vi "Main_PXI_v1.0.vi"() -> ()   [LabVIEW 2018]
doc: "Main VI for the controls"
uses:
  components/pmcl dynamic signal analyzer/Controls/DSA excitation specs.ctl
  components/pmcl dynamic signal analyzer/Controls/DSA cycle specs.ctl
  Typedefs/StateDef_Enum.ctl
  <vilib>/Simulation/Scripting/Companion Diagram/SimConfigNode/SimParams.ctl
  <vilib>/Simulation/Scripting/Companion Diagram/SimConfigNode/_simSolvers.ctl
  <vilib>/Simulation/Implementation/Shared/SIMSCR Execution Mode.ctl
  <vilib>/Platform/TimedLoop/XDataNode/timing_clust.ctl
  <vilib>/Platform/TimedLoop/XDataNode/nitl_modes.ctl
  <vilib>/Platform/TimedLoop/XDataNode/wakeup.ctl
  <vilib>/Simulation/Param Hierarchy/Typedefs/SIMPH Param Control Actions.ctl
  <vilib>/Simulation/Implementation/Shared/SIM limit type.ctl
  <vilib>/Simulation/Scripting/Editor Utilities/SIM subVI tag data.ctl
  <vilib>/Simulation/Scripting/Editor Utilities/SIM subVI execution type.ctl
  <vilib>/Simulation/Implementation/Shared/NILVSim_ParamChanged.vi
  <vilib>/Simulation/Implementation/Shared/NILVSim_FinishedLate.vi
  <vilib>/Simulation/Implementation/Shared/NILVSIM_BeginStep.vi
  <vilib>/DAQmx/read.llb/DAQmx Read.vi
  <vilib>/DAQmx/read.llb/DAQmx Read (Analog 1D DBL NChan 1Samp).vi
  <vilib>/Simulation/Utility/Implementation/SIM SimulationParams.vi
  <vilib>/Simulation/ContinuousLinear/Implementation/NILVSim Integrator new.llb/SIM Integrator distributor (scalar).vi
  <vilib>/Simulation/Implementation/Shared/SIM Fire Discrete SubVI.vi
  <vilib>/Simulation/ContinuousLinear/Implementation/NILVSim Transfer Function Direct.llb/SIM Transfer Function Direct (SISO).vi
  <vilib>/DAQmx/write.llb/DAQmx Write (Analog DBL 1Chan 1Samp).vi
  <vilib>/Simulation/Utility/Implementation/SIM Halt.vi
  <vilib>/Simulation/SignalArithmetic/Implementation/NILVSim Gain.llb/SIM Gain (scalar).vi
  <vilib>/Simulation/ContinuousLinear/Implementation/NILVSim Integrator new.llb/SIM Integrator collector (scalar).vi
  <vilib>/Simulation/Implementation/Shared/NILVSim_Manager.vi
  <vilib>/Utility/error.llb/Clear Errors.vi
  <vilib>/Simulation/Implementation/Shared/NILVSim_FinalizeModel.vi
  <vilib>/Simulation/Utility/Implementation/NILVSim SimulationParams (core).vi
  <vilib>/Simulation/Implementation/Shared/SIM Fire Discrete SubVI (Core).vi
  <vilib>/DAQmx/create/channels.llb/DAQmx Create Channel (AO-Voltage-Basic).vi
  <vilib>/DAQmx/create/channels.llb/DAQmx Create Channel (AI-Voltage-Basic).vi
  <vilib>/Simulation/Implementation/Shared/SIM Unbundle Sim Info.vi
  <vilib>/Simulation/Implementation/Shared/SIMSH Read Queue.vi
  <vilib>/Simulation/Implementation/Shared/NILVSim_Initialize.vi
  <vilib>/DAQmx/miscellaneous.llb/DAQmx Fill In Error Info.vi
  <vilib>/Simulation/Utility/Implementation/NILVSim Get Time and IsAcceptedStep.vi
  <vilib>/Simulation/Implementation/Shared/NILVSim_GetModelError.vi
  <vilib>/Simulation/Implementation/Shared/SIM Bundle Sim Info.vi
  <vilib>/Simulation/Scripting/Companion Diagram/SimConfigNode/SimDog.xnode
  <vilib>/Platform/TimedLoop/XDataNode/XDataNode.xnode
  <vilib>/Simulation/Implementation/XNodeFramework/SimXNode/SimX.xnode
  Components/Timing/Timing.lvlib
  <vilib>/Platform/TimedLoop/XDataNode/XDNodeRunTimeDep.lvlib
  <vilib>/Analysis/NI_AALPro.lvlib
  <vilib>/ptbypt/NI_PtbyPt.lvlib
  <vilib>/Simulation/ContinuousLinear/Implementation/NILVSim Integrator new.llb/SIM Integrator (scalar).vi
  <vilib>/Simulation/Implementation/Shared/NI_SIM_Implementation.lvlib
panel:
  in  "System Stop Button":bool
  in  "Pause chart?":bool
  in  "Controller Params":enum32{"Page 1"}(tab)
  in  "Kp":dbl=1.0 min=0.0
  in  "Controller On?":bool
  out "Status":string
  in  "Ref. Gen.":enum32{"Analog In", "Manual", "Wave Gen", "DSA"}(tab)=enum."Wave Gen"
  in  "Ref. cmd.":dbl(slide) step=1.0 scale=-10.0..10.0 scale format="%#.1f"
  in  "Signal Cluster":T1={"phase"=0.0, "amplitude"=1.0, "frequency"=1.0, "offset"=1.0, "Signal"=enum."Square"} {"offset" format="%0.2f"; "frequency" format="%0.2f"; "amplitude" format="%0.2f"; "phase" format="%0.2f"}
  in  "Frequency\nResponse":enum16{"Plant", "RR", "CL"}(ring)
  out "DSA \nRunning?":bool
  in  "Stop \nDSA":bool
  in  "Start \nDSA":bool
  in  "DSA excitation specs":T2={"Initial Freq. [Hz]"=10.0, "Final Freq. [Hz]"=999.0, "# pts. in interval"=50, "Samping Time [s]"=0.001, "Amplitude [V]"=1.0, "Offset [V]"=0.0, "Freq Units (F: rad/s, T: Hz)"=TRUE}
  in  "Cycle Specs":T3={"Cycles To \nSettle (M)"=5, "Cycles To \nCalculate (N)"=10}
  in  "Loop Timing":enum32{"CD&Sim", "Ref. gen", "UI"}(tab)
  out "# Finished\nLate counter":dbl
  in  "CD&Sim\nLoop Rate (Hz)":dbl=10000.0 format="%#_4p"
  out "# Finished\nLate counter":dbl
  in  "Ref. Gen.\nLoop Rate (Hz)":dbl=10000.0 format="%#_4p"
  in  "UI Loop rate (Hz)":dbl=1000.0 format="%#_6p"
  in  "Display Waveforms":enum32{"Controller Signals", "DSA "}(tab)
  out "Control Effort":dbl(graph)
  out "Waveform Chart":cluster{"Double":dbl, "Numeric":dbl}(graph)
  out "Phase Bode Plot":cluster{dbl[], dbl[]}(graph)
  out "Magnitude Bode Plot":cluster{dbl[], dbl[]}(graph)
  out "DSA Signals":cluster{"Double":dbl, "Double":dbl}(graph)
  # "Connect the Reference Signal \nto C/AI 1 of the myRIO."
  # "Pinout Config.:\nPort C/AI0 : Plant output being read           by the myRIO.\nPort C/AI1 : Reference signal for the control loop.\nPort C/AO0 : Control effort signal to the plant."
  # "Control Loop Timing"
  # "Ref.  Gen. Loop Timing"
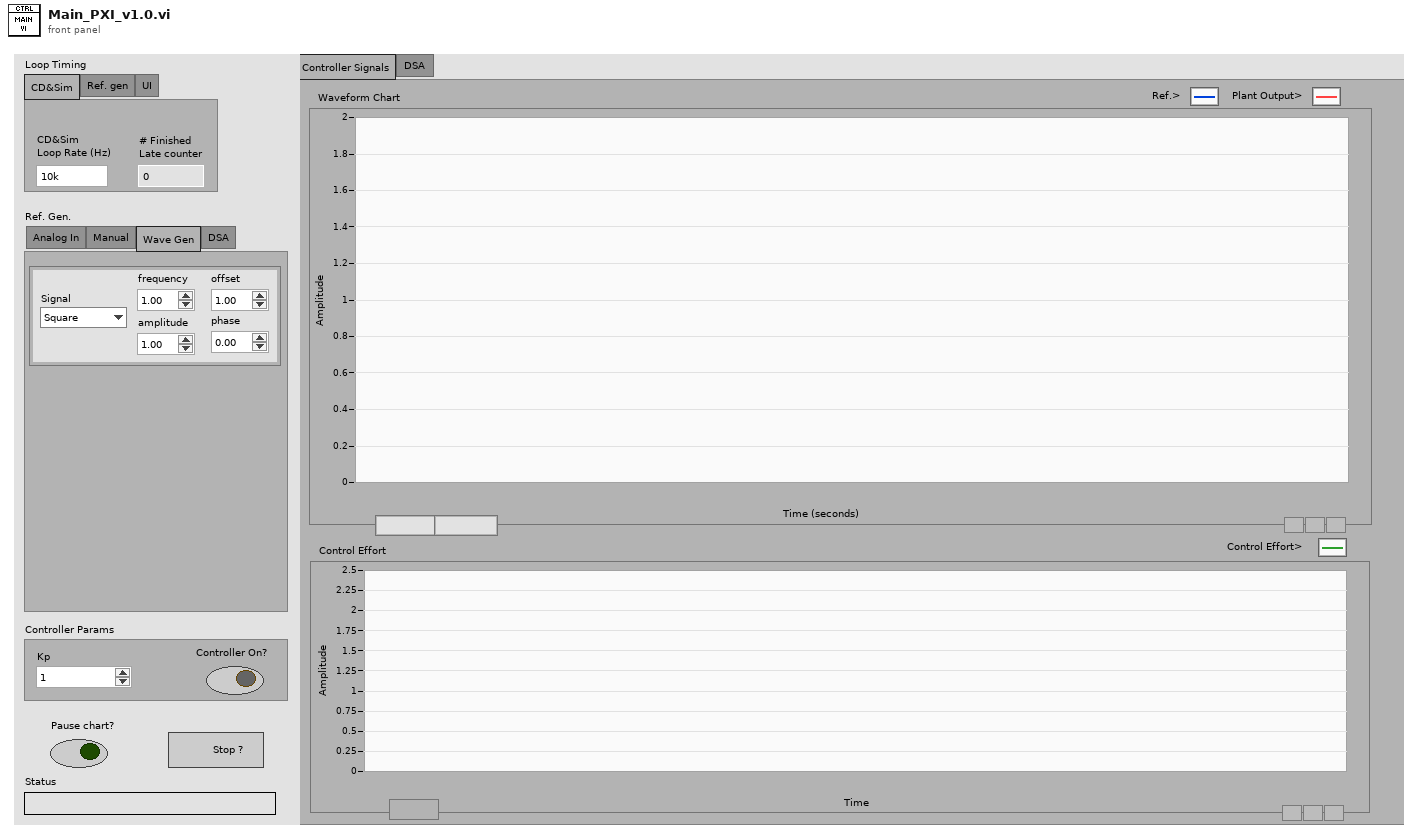
[diagram p1: front panel]
types:
  T1 = cluster{"phase":dbl, "amplitude":dbl, "frequency":dbl, "offset":dbl, "Signal":enum16{"Sine", "Square", "Sawtooth"}}
  T2 = typedef "DSA excitation specs.ctl" = cluster{"Initial Freq. [Hz]":dbl, "Final Freq. [Hz]":dbl, "# pts. in interval":i16, "Samping Time [s]":dbl, "Amplitude [V]":dbl, "Offset [V]":dbl, "Freq Units (F: rad/s, T: Hz)":bool}
  T3 = typedef "DSA cycle specs.ctl" = cluster{"Cycles To \nSettle (M)":i16, "Cycles To \nCalculate (N)":i16}
  T4 = typedef "StateDef_Enum.ctl" = enum16{"Initialize", "Wait", "Shutdown"}
  T5 = typedef "XDNodeRunTimeDep.lvlib/timing_clust.ctl" = cluster{"Expected End [f-1]":u64, "Actual End [f-1]":u64, "Finished Late? [f-1]":bool, "Expected End [i-1]":u64, "Actual End [i-1]":u64, "Finished Late? [i-1]":bool, "Expected Start [i]":u64, "Actual Start [i]":u64, "Expected Start [f]":u64, "Actual Start [f]":u64, "Source Name":string, "Structure Name":string, "Period":i64, "Deadline":i64, "Offset":i64, "Start":i64, "Priority":i32, "Timeout":i32, "Mode":T6, "Wakeup Reason":T7, "Error":errorcluster, "Source Type":string, "Secondary Source Type":string, "Global End Time":u64, "Global Start Time":u64, "Frame Duration":u64, "Iteration Duration":u64, "Assigned CPU":i32, "I/O Scan Engine Mode":u32}
  T6 = typedef "XDNodeRunTimeDep.lvlib/nitl_modes.ctl" = enum32{"No Change", "Process missed periods, maintain original phase", "Discard missed periods, maintain original phase", "Process missed periods, ignore original phase", "Discard missed periods, ignore original phase"}
  T7 = typedef "XDNodeRunTimeDep.lvlib/wakeup.ctl" = enum32{"Normal", "Aborted", "Asynchronous wakeup", "Timing source error", "Timed loop error", "Timeout"}
  T8 = cluster{"Analog In CH1":dbl, "Analog In CH0":dbl}
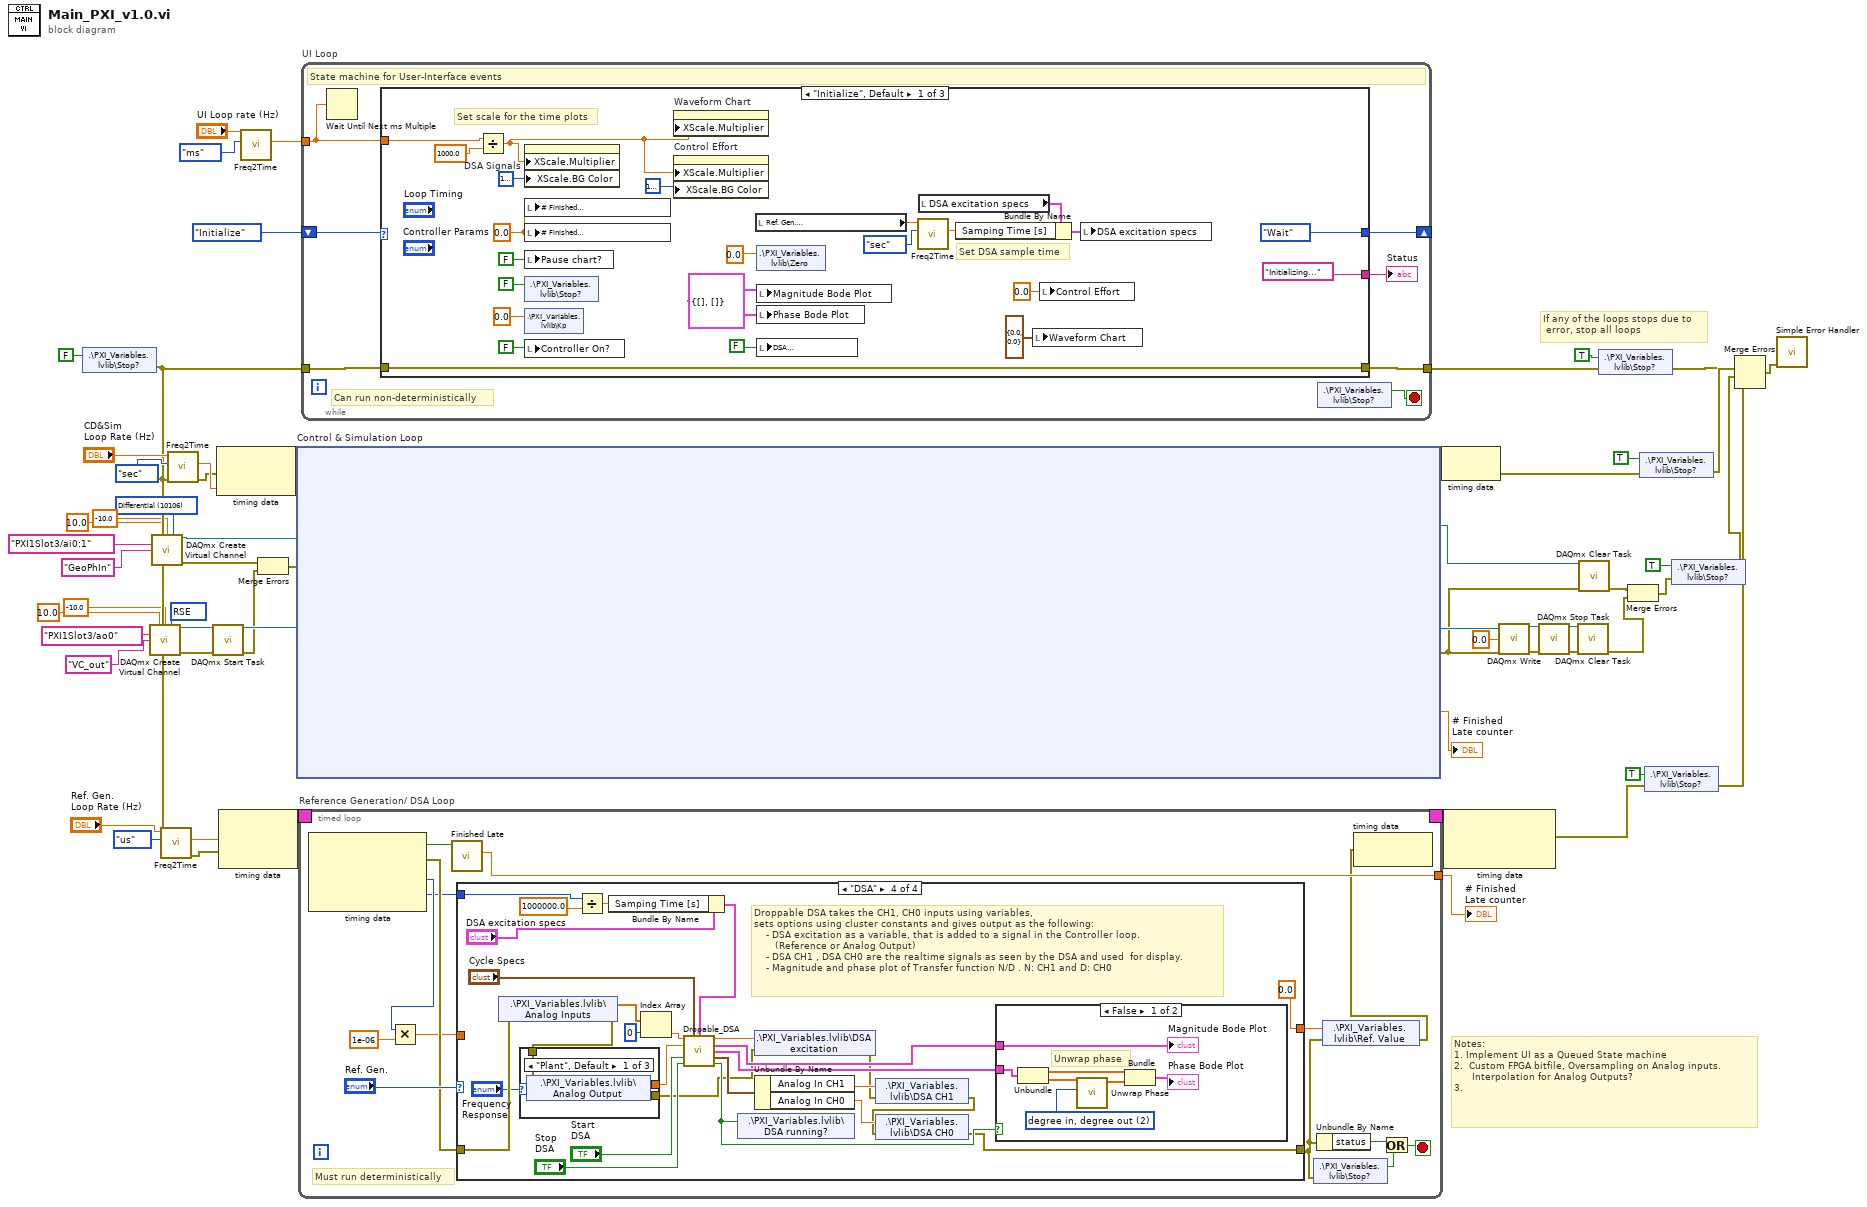
[diagram p0: block diagram]
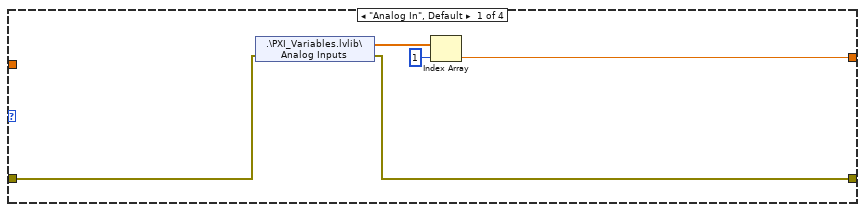
[diagram p2: hidden frame]
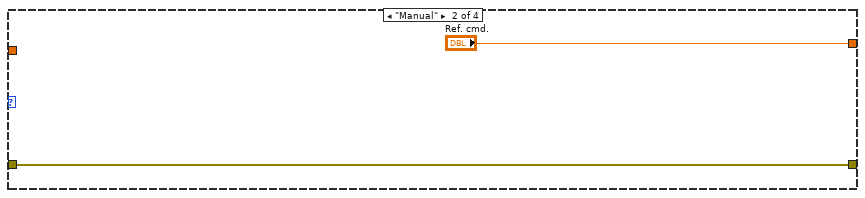
[diagram p3: hidden frame]
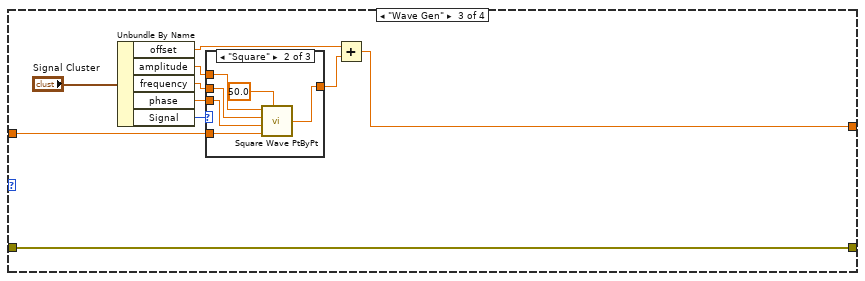
[diagram p4: hidden frame]
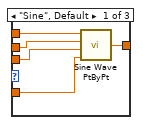
[diagram p5: hidden frame]
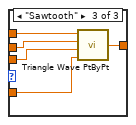
[diagram p6: hidden frame]
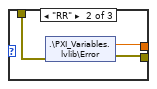
[diagram p7: hidden frame]
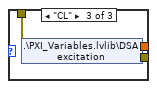
[diagram p8: hidden frame]
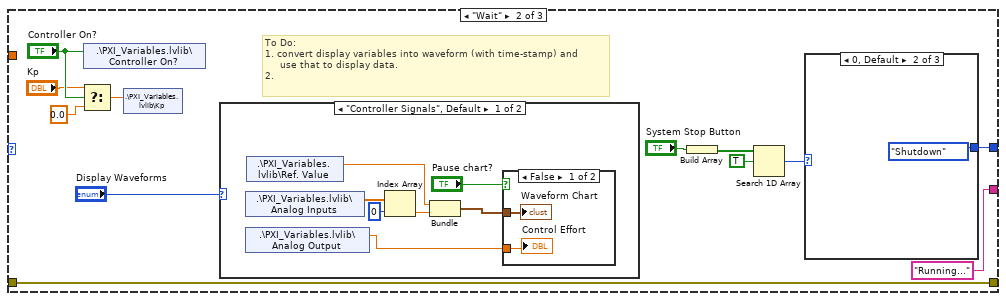
[diagram p10: hidden frame]
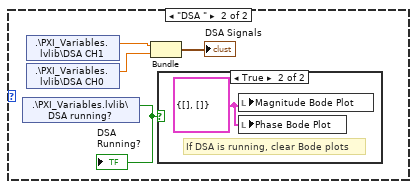
[diagram p12: hidden frame]
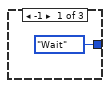
[diagram p14: hidden frame]
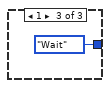
[diagram p15: hidden frame]
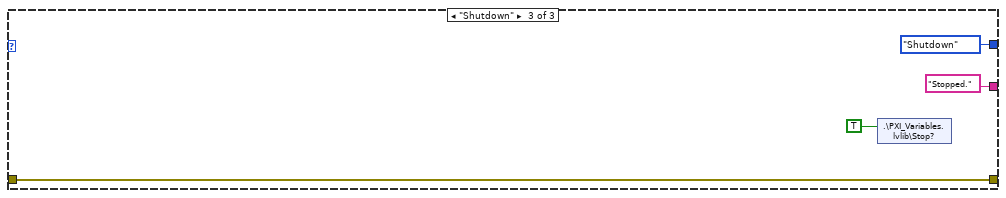
[diagram p16: hidden frame]
diagram:
  w9 = 10106 items=["Default"=-1, "RSE"=10083, "NRSE"=10078, "Differential"=10106, "Pseudodifferential"=12529] ("input terminal configuration")
  w23 = 10083 items=["Default"=-1, "RSE"=10083, "Differential"=10106, "Pseudodifferential"=12529] ("output terminal configuration")
  # "Notes:\n1. Implement UI as a Queued State machine\n2.  Custom FPGA bitfile, Oversampling on Analog inputs. \n      Interpolation for Analog Outputs?\n3."
  # "If any of the loops stops due to\n error, stop all loops"
  n1 = shared-variable ".\\PXI_Variables.lvlib\\Stop?"(FALSE ("Stop?")) -> (error out=w30:errorcluster)  [unwired: 1 in]
  n2 = call-poly <vilib>:"DAQmx Create Virtual Channel.vi"("maximum value"=10.0, "minimum value"=-10.0, "output terminal configuration"=w23, "physical channels"=tag "PXI1Slot3/ao0", "name to assign"="VC_out") -> ("task out"=w21:refnum<k21>, "error out"=w20:errorcluster)  [unwired: 9 in]
  n3 = call-poly <vilib>:"DAQmx Create Virtual Channel.vi"("maximum value"=10.0, "minimum value"=-10.0, "input terminal configuration"=w9, "physical channels"=tag "PXI1Slot3/ai0:1", "name to assign"="GeoPhIn") -> ("task out"=w4:refnum<k21>, "error out"=w5:errorcluster)  [unwired: 9 in]
  n4 = call "Freq2Time.vi"("error in (no error)"=w30, "Int. Time Unit"=enum16{"sec", "us", "ms"}."us", "Sample rate (Hz)"="Ref. Gen.\nLoop Rate (Hz)") -> ("error out"=w44:errorcluster, "Int.  time [unit]"=w48:dbl)  [unwired: 6 in, 1 out]
  n5 = call "Freq2Time.vi"("error in (no error)"=w30, "Int. Time Unit"=enum16{"sec", "us", "ms"}."sec", "Sample rate (Hz)"="CD&Sim\nLoop Rate (Hz)") -> ("error out"=w45:errorcluster, "Int.  time [unit]"=w55:dbl)  [unwired: 6 in, 1 out]
  n6 = call <vilib>:"DAQmx Start Task.vi"("task/channels in"=w21, "error in"=w20) -> ("task out"=w19:refnum<k21>, "error out"=w18:errorcluster)  [unwired: 12 in]
  n7 = node-c288(w45, w55) -> (w59:variant)
  n8 = node-c288(w48, w44) -> (w51:T5)
  n9 = call "Freq2Time.vi"("Int. Time Unit"=enum16{"sec", "us", "ms"}."ms", "Sample rate (Hz)"="UI Loop rate (Hz)") -> ("Int.  time [unit]"=w35:dbl)  [unwired: 7 in, 2 out]
  n10 = Merge Errors(w5, w18) -> (w52:errorcluster)
  n11 = node-c254 "Control & Simulation Loop"(w59, w52, w19, w4) -> (w58:variant, →"# Finished\nLate counter":dbl, w17:refnum<k21>, w3:errorcluster, w1:refnum<k21>)
  n12 = timed-loop "Reference Generation/ DSA Loop" {
    timing: w51 -> [_]
    timing-out: [_] -> w50
    tunnel: [w73] -> w46
    stop <- w67 stop-if-true
    # "Must run deterministically"
    n13 = node-c288() -> (w74:bool, w70:errorcluster, w64:i64, w63:i64)  [unwired: 1 in]
    n14 = Multiply(x=w64, y=1e-06) -> (x*y=w66:dbl)
    n15 = call "Finished Late.vi"("Finished \nLate?"=w74) -> ("# Finished\nLate counter"=w73:dbl)  [unwired: 8 in, 2 out]
    n16 = case shown="\"DSA\"" "Ref. Gen." {
      tunnel: [w79 "Ref. cmd." w84 0.0 ("Ref. cmd.")] -> w71
      tunnel: w70 -> [w77 w80 w83 w114]
      tunnel: [w76 w80 w83 w117] -> w61
      tunnel: w66 -> [_ _ w82 _]
      tunnel: w63 -> [_ _ _ w124]
      frame "Analog In", Default {
        n17 = shared-variable ".\\PXI_Variables.lvlib\\Analog Inputs"(error in=w77) -> (w78:dbl[], error out=w76:errorcluster)
        n18 = Index Array(array=w78, index=1) -> (element=w79:dbl)
      }
      frame "Manual" {
      }
      frame "Wave Gen" {
        n19 = Unbundle By Name("Signal Cluster") -> ("offset"=w85:dbl, "amplitude"=w88:dbl, "frequency"=w87:dbl, "phase"=w86:dbl, "Signal"=w89:enum16{"Sine", "Square", "Sawtooth"})
        n20 = case shown="\"Square\"" w89 {
          tunnel: [w96 w101 w107] -> w91
          tunnel: w88 -> [w95 w100 w106]
          tunnel: w87 -> [w94 w99 w105]
          tunnel: w86 -> [w93 w98 w104]
          tunnel: w82 -> [w92 w97 w103]
          frame "Sine", Default {
            n21 = call <vilib>:"Sine Wave PtByPt.vi"("time"=w92, "phase"=w93, "frequency"=w94, "amplitude"=w95) -> ("sine wave"=w96:dbl)
          }
          frame "Square" {
            n22 = call <vilib>:"Square Wave PtByPt.vi"("amplitude"=w100, "frequency"=w99, "phase"=w98, "time"=w97, "duty cycle (%)"=50.0) -> ("square wave"=w101:dbl)
          }
          frame "Sawtooth" {
            n23 = call <vilib>:"Triangle Wave PtByPt.vi"("time"=w103, "phase"=w104, "frequency"=w105, "amplitude"=w106) -> ("triangle wave"=w107:dbl)
          }
        }
        n24 = Add(x=w85, y=w91) -> (x+y=w84:dbl)
      }
      frame "DSA" {
        # "Droppable DSA takes the CH1, CH0 inputs using variables, \nsets options using cluster constants and gives output as the following:\n    - DSA excitation as a variable, that is added to a signal in the Controller loop. \n       (Reference or Analog Output)\n    - DSA CH1 , DSA CH0 are the realtime signals as seen by the DSA and used  for display.\n    - Magnitude and phase plot of Transfer function N/D . N: CH1 and D: CH0"
        n25 = shared-variable ".\\PXI_Variables.lvlib\\Analog Inputs"(error in=w114) -> (w113:dbl[], error out=w111:errorcluster)
        n26 = case shown="\"Plant\", Default" "Frequency\nResponse" {
          tunnel: [w137 w140 w141] -> w112
          tunnel: w111 -> [w136 w138 w143]
          tunnel: [w135 w139 w142] -> w108
          frame "Plant", Default {
            n27 = shared-variable ".\\PXI_Variables.lvlib\\Analog Output"(error in=w136) -> (w137:dbl, error out=w135:errorcluster)
          }
          frame "RR" {
            n28 = shared-variable ".\\PXI_Variables.lvlib\\Error"(error in=w138) -> (w140:dbl, error out=w139:errorcluster)
          }
          frame "CL" {
            n29 = shared-variable ".\\PXI_Variables.lvlib\\DSA excitation"(error in=w143) -> (w141:dbl, error out=w142:errorcluster)
          }
        }
        n30 = Divide(x=w124, y=1000000.0) -> (x/y=w122:dbl)
        n31 = Bundle By Name(cluster="DSA excitation specs", "Samping Time [s]"=w122) -> (w121:T2)
        n32 = Index Array(array=w113, index=0) -> (element=w115:dbl)
        n33 = call "Dropable_DSA.vi"("Analog In CH1"=w115, "Cycle Specs"="Cycle Specs", "Excitation Specs"=w121, "Analog In CH0"=w112, "START"="Start \nDSA", "STOP"="Stop \nDSA") -> ("Analog Out"=w133:dbl, "Bode Magnitude"=w126:cluster{dbl[], dbl[]}, "Bode Phase"=w125:cluster{dbl[], dbl[]}, "Live signals"=w130:T8, "Running"=w120:bool)  [unwired: 4 in, 1 out]
        n34 = shared-variable ".\\PXI_Variables.lvlib\\DSA running?"(w120) -> ()  [unwired: 1 in, 1 out]
        n35 = shared-variable ".\\PXI_Variables.lvlib\\DSA excitation"(w133, error in=w108) -> (error out=w119:errorcluster)
        n36 = Unbundle By Name(w130) -> ("Analog In CH1"=w129:dbl, "Analog In CH0"=w128:dbl)
        n37 = shared-variable ".\\PXI_Variables.lvlib\\DSA CH1"(w129, error in=w119) -> (error out=w118:errorcluster)
        n38 = shared-variable ".\\PXI_Variables.lvlib\\DSA CH0"(w128, error in=w118) -> (error out=w117:errorcluster)
        n39 = case shown="False" w120 {
          tunnel: w126 -> [w144 _]
          tunnel: w125 -> [w146 _]
          frame False {
            w148 = 2 items=["radian in, radian out", "radian in, degree out", "degree in, degree out", "degree in, radian out"] ("phase unit")
            # "Unwrap phase"
            n40 = Unbundle(w146) -> (w150:dbl[], w147:dbl[])
            n41 = call <vilib>:"Unwrap Phase.vi"("phase unit"=w148, "Phase"=w147) -> ("Unwrapped Phase"=w149:dbl[])  [unwired: 8 in, 1 out]
            n42 = Bundle(w150, "Unwrapped Phase"=w149) -> (→"Phase Bode Plot":cluster{dbl[], "Unwrapped Phase":dbl[]})  [unwired: 1 in]
            "Magnitude Bode Plot" <- w144
          }
          frame True {
          }
        }
      }
    }
    n43 = shared-variable ".\\PXI_Variables.lvlib\\Stop?"(error in=w61) -> (w68:bool)  [unwired: 1 out]
    n44 = Unbundle By Name(w61) -> ("status"=w69:bool)
    n45 = shared-variable ".\\PXI_Variables.lvlib\\Ref. Value"(w71, error in=w61) -> (error out=w62:errorcluster)
    n46 = node-c288(w62) -> ()  [unwired: 1 out]
    n47 = Or(x=w69, y=w68) -> (x .or. y?=w67:bool)
  }
  "# Finished\nLate counter" <- w46
  n48 = while "UI Loop" {
    shift-right: [w164] -> _
    shift-left: StateDef_Enum."Initialize" ("State defining Enum") -> [w165]
    tunnel: w30 -> [w163]
    tunnel: [w162] -> w34
    tunnel: w35 -> [w159]
    stop <- w160 stop-if-true
    # "Can run non-deterministically"
    # "State machine for User-Interface events"
    n49 = Wait Until Next ms Multiple(millisecond multiple=w159) -> ()  [unwired: 1 out]
    n50 = case shown="\"Initialize\", Default" w165 {
      tunnel: [StateDef_Enum."Wait" ("State defining Enum") w197 StateDef_Enum."Shutdown" ("State defining Enum")] -> w164
      tunnel: w163 -> [w185 w195 w221]
      tunnel: [w185 w195 w221] -> w162
      tunnel: ["Initializing..." ("Status") "Running..." ("Status") "Stopped." ("Status")] -> w161
      tunnel: w159 -> [w183 _ _]
      frame "Initialize", Default {
        w177 = cluster{dbl[], dbl[]} {[], []} ("Magnitude Bode Plot")
        w179 = 0.0 ("# Finished\nLate counter")
        # "Set DSA sample time"
        # "Set scale for the time plots"
        n51 = Divide(x=w183, y=1000.0) -> (x/y=w169:dbl)
        n52 = property on="DSA Signals" class="WFChart (strict)"("XScale.Multiplier"=w169, "XScale.BG Color"=u32 16777216) -> ()  [unwired: 2 in, 2 out]
        n53 = local write "# Finished\nLate counter"(w179) -> ()
        n54 = local write "# Finished\nLate counter"(w179) -> ()
        n55 = local write "Pause chart?"(FALSE ("Pause chart?")) -> ()
        n56 = shared-variable ".\\PXI_Variables.lvlib\\Stop?"(FALSE ("Stop?")) -> ()  [unwired: 1 in, 1 out]
        n57 = shared-variable ".\\PXI_Variables.lvlib\\Kp"(0.0 ("Kp")) -> ()  [unwired: 1 in, 1 out]
        n58 = local write "Controller On?"(FALSE ("Controller On?")) -> ()
        n59 = property on="Waveform Chart" class="WFChart (strict)"("XScale.Multiplier"=w169) -> ()  [unwired: 2 in, 2 out]
        n60 = property on="Control Effort" class="WFChart (strict)"("XScale.Multiplier"=w169, "XScale.BG Color"=u32 16777216) -> ()  [unwired: 2 in, 2 out]
        n61 = local read "Ref. Gen.\nLoop Rate (Hz)"() -> (w172:dbl)
        n62 = shared-variable ".\\PXI_Variables.lvlib\\Zero"(0.0 ("Zero")) -> ()  [unwired: 1 in, 1 out]
        n63 = local write "Magnitude Bode Plot"(w177) -> ()
        n64 = local write "Phase Bode Plot"(w177) -> ()
        n65 = local write "DSA \nRunning?"(FALSE ("DSA \nRunning?")) -> ()
        n66 = call "Freq2Time.vi"("Int. Time Unit"=enum16{"sec", "us", "ms"}."sec", "Sample rate (Hz)"=w172) -> ("Int.  time [unit]"=w170:dbl)  [unwired: 7 in, 2 out]
        n67 = local read "DSA excitation specs"() -> (w174:T2)
        n68 = Bundle By Name(cluster=w174, "Samping Time [s]"=w170) -> (w173:T2)
        n69 = local write "Waveform Chart"(cluster{"Double":dbl, "Numeric":dbl} {"Double"=0.0, "Numeric"=0.0} ("Waveform Chart")) -> ()
        n70 = local write "Control Effort"(0.0 ("Control Effort")) -> ()
        n71 = local write "DSA excitation specs"(w173) -> ()
      }
      frame "Wait" {
        # "To Do:\n1. convert display variables into waveform (with time-stamp) and\n     use that to display data.\n2."
        n72 = Select(t="Kp", s="Controller On?", f=0.0) -> (s? t:f=w193:dbl)
        n73 = shared-variable ".\\PXI_Variables.lvlib\\Controller On?"("Controller On?") -> ()  [unwired: 1 in, 1 out]
        n74 = shared-variable ".\\PXI_Variables.lvlib\\Kp"(w193) -> ()  [unwired: 1 in, 1 out]
        n75 = case shown="\"Controller Signals\", Default" "Display Waveforms" {
          frame "Controller Signals", Default {
            n76 = shared-variable ".\\PXI_Variables.lvlib\\Analog Inputs"() -> (w207:dbl[])  [unwired: 1 in, 1 out]
            n77 = shared-variable ".\\PXI_Variables.lvlib\\Analog Output"() -> (w201:dbl)  [unwired: 1 in, 1 out]
            n78 = shared-variable ".\\PXI_Variables.lvlib\\Ref. Value"() -> (w204:dbl)  [unwired: 1 in, 1 out]
            n79 = Index Array(array=w207, index=0) -> (element=w206:dbl)
            n80 = Bundle("Double"=w204, "Numeric"=w206) -> (w202:cluster{"Double":dbl, "Numeric":dbl})  [unwired: 1 in]
            n81 = case shown="False" "Pause chart?" {
              tunnel: w202 -> [w209 _]
              tunnel: w201 -> [w208 _]
              frame False {
                "Waveform Chart" <- w209
                "Control Effort" <- w208
              }
              frame True {
              }
            }
          }
          frame "DSA " {
            n82 = shared-variable ".\\PXI_Variables.lvlib\\DSA running?"() -> (w210:bool)  [unwired: 1 in, 1 out]
            "DSA \nRunning?" <- w210
            n83 = shared-variable ".\\PXI_Variables.lvlib\\DSA CH1"() -> (w212:dbl)  [unwired: 1 in, 1 out]
            n84 = shared-variable ".\\PXI_Variables.lvlib\\DSA CH0"() -> (w211:dbl)  [unwired: 1 in, 1 out]
            n85 = Bundle("Double"=w212, "Double"=w211) -> (→"DSA Signals":cluster{"Double":dbl, "Double":dbl})  [unwired: 1 in]
            n86 = case shown="True" w210 {
              frame False {
              }
              frame True {
                w214 = cluster{dbl[], dbl[]} {[], []} ("Magnitude Bode Plot")
                # "If DSA is running, clear Bode plots"
                n87 = local write "Magnitude Bode Plot"(w214) -> ()
                n88 = local write "Phase Bode Plot"(w214) -> ()
              }
            }
          }
        }
        n89 = Build Array("System Stop Button") -> (w199:bool[])
        n90 = Search 1D Array(1D array=w199, element=TRUE) -> (index of element=w196:i32)  [unwired: 1 in]
        n91 = case shown="0, Default" w196 {
          tunnel: [StateDef_Enum."Wait" ("State defining Enum") StateDef_Enum."Shutdown" ("State defining Enum") StateDef_Enum."Wait" ("State defining Enum")] -> w197
          frame -1 {
          }
          frame 0, Default {
          }
          frame 1 {
          }
        }
      }
      frame "Shutdown" {
        n92 = shared-variable ".\\PXI_Variables.lvlib\\Stop?"(TRUE) -> ()  [unwired: 1 in, 1 out]
      }
    }
    "Status" <- w161
    n93 = shared-variable ".\\PXI_Variables.lvlib\\Stop?"() -> (w160:bool)  [unwired: 1 in, 1 out]
  }
  n94 = node-c288(w58) -> (w43:errorcluster)
  n95 = node-c288(w50) -> (w40:errorcluster)  [unwired: 1 out]
  n96 = call-poly <vilib>:"DAQmx Write.vi"("task/channels in"=w17, "data"=0.0, "error in"=w3) -> ("task out"=w15:refnum<k21>, "error out"=w14:errorcluster)  [unwired: 10 in, 1 out]
  n97 = call <vilib>:"DAQmx Stop Task.vi"("task/channels in"=w15, "error in"=w14) -> ("task out"=w13:refnum<k21>, "error out"=w12:errorcluster)  [unwired: 12 in]
  n98 = call <vilib>:"DAQmx Clear Task.vi"("task in"=w13, "error in"=w12) -> ("error out"=w11:errorcluster)  [unwired: 13 in]
  n99 = call <vilib>:"DAQmx Clear Task.vi"("task in"=w1, "error in"=w3) -> ("error out"=w2:errorcluster)  [unwired: 13 in]
  n100 = shared-variable ".\\PXI_Variables.lvlib\\Stop?"(TRUE ("Stop?"), error in=w34) -> (error out=w33:errorcluster)
  n101 = Merge Errors(w2, w11) -> (w28:errorcluster)
  n102 = shared-variable ".\\PXI_Variables.lvlib\\Stop?"(TRUE ("Stop?"), error in=w43) -> (error out=w42:errorcluster)
  n103 = shared-variable ".\\PXI_Variables.lvlib\\Stop?"(TRUE ("Stop?"), error in=w40) -> (error out=w39:errorcluster)
  n104 = shared-variable ".\\PXI_Variables.lvlib\\Stop?"(TRUE ("Stop?"), error in=w28) -> (error out=w27:errorcluster)
  n105 = Merge Errors(w33, w42, w27, w39) -> (w53:errorcluster)
  n106 = call <vilib>:"Simple Error Handler.vi"("error in (no error)"=w53) -> ()  [unwired: 4 in, 5 out]
